vi "写自测概述.vi"(8 "合格路数":i32, 9 "共路数":i32, 10 "测试事项":string, 11 "自测序号":i32) -> (2 "概述字符串":string)   [LabVIEW 2010]
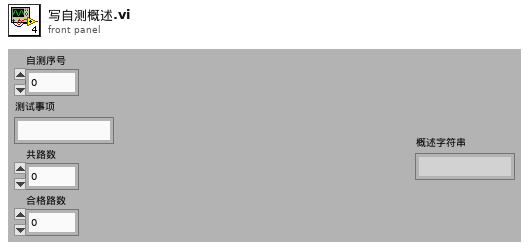
[diagram p1: front panel]
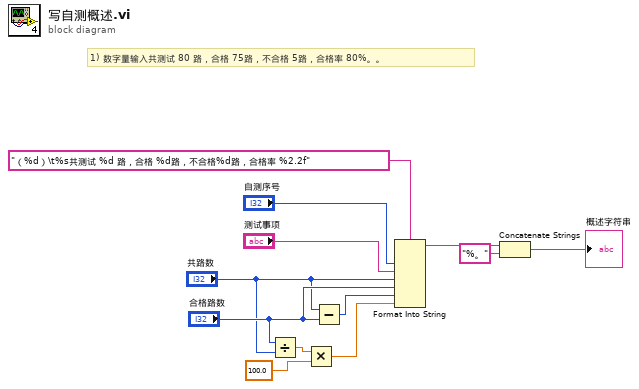
[diagram p0: block diagram]
diagram:
  # "1)\t数字量输入共测试 80 路，合格 75路，不合格 5路，合格率 80%。。"
  n1 = Divide(x="合格路数", y="共路数") -> (x/y=w6:dbl)
  n2 = Multiply(x=w6, y=100.0) -> (x*y=w4:dbl)
  n3 = Subtract(x="共路数", y="合格路数") -> (x-y=w9:i32)
  n4 = Format Into String(format string="（%d）\t%s共测试 %d 路，合格 %d路，不合格%d路，合格率 %2.2f", "自测序号", "测试事项", "共路数", "合格路数", w9, w4) -> (resulting string=w3:string)  [unwired: 2 in, 1 out]
  n5 = Concatenate Strings(w3, "%。" ("字符串")) -> (→"概述字符串":string)
